vi "MainFGV.vi"(7 "FGV_mods":T1, 8 "Error In":errorcluster, 11 "DataIn":variant) -> (0 "Error Out":errorcluster, 3 "DataOut":variant)   [LabVIEW 2016]
uses:
  MainFGV_mods.ctl
  Log/log_mods.ctl
  Log/log_status.ctl
  <vilib>/DAQmx/read.llb/DAQmx Read (Analog 2D DBL NChan NSamp).vi
  <vilib>/DAQmx/miscellaneous.llb/DAQmx Fill In Error Info.vi
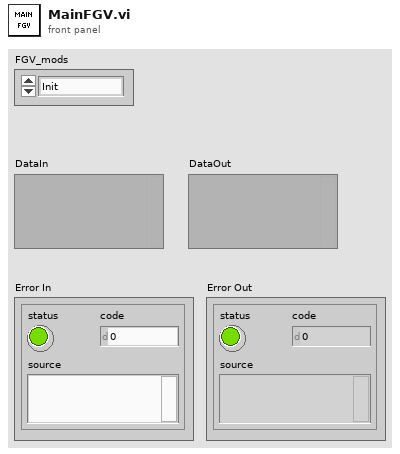
[diagram p1: front panel]
types:
  T1 = typedef "MainFGV_mods.ctl" = enum16{"Init", "Config", "Advanced", "CreateTask", "Register", "Acquire", "Start", "Burst", "Record", "End"}
  T2 = typedef "log_mods.ctl" = enum16{"Init", "LogFileRefnum", "SetStatus", "WriteAcel", "WriteToLog", "End"}
  T3 = typedef "log_status.ctl" = enum16{"Init", "Ready", "Running", "Error", "End"}
  T4 = typedef "MainFGV_data.ctl" = cluster{"TestDir":path, "TestName":string, "task":refnum<k21>, "data_file":refnum<file>, "burts_file":refnum<file>, "log_file":refnum<file>, "SamplesPerChannel":dbl, "AcqQueue":refnum<queue>, "StartTime":timestamp, "config_channels":T5[], "DAQmx Device":tag, "Advanced":T6}
  T5 = typedef "config_board.ctl" = cluster{"Sens 1":dbl, "active 1":bool, "type 1":bool, "type 2":bool, "active 2":bool, "Sens 2":dbl, "type 3":bool, "active 3":bool, "Sens 3":dbl, "type 4":bool, "active 4":bool, "Sens 4":dbl}
  T6 = typedef "AdvancedConfig.ctl" = cluster{"rate":dbl, "duration":dbl, "thr":dbl, "preTrigger":dbl, "cutoff":dbl, "Filtro":enum16{"Desativado", "Passa banda", "Passa alta", "Passa baixa"}, "highPass":dbl, "lowPass":dbl}
  T7 = cluster{"seconds since 1Jan1904":timestamp, dbl[]}
  T8 = cluster{"seconds since 1Jan1904":timestamp, dbl[][]}
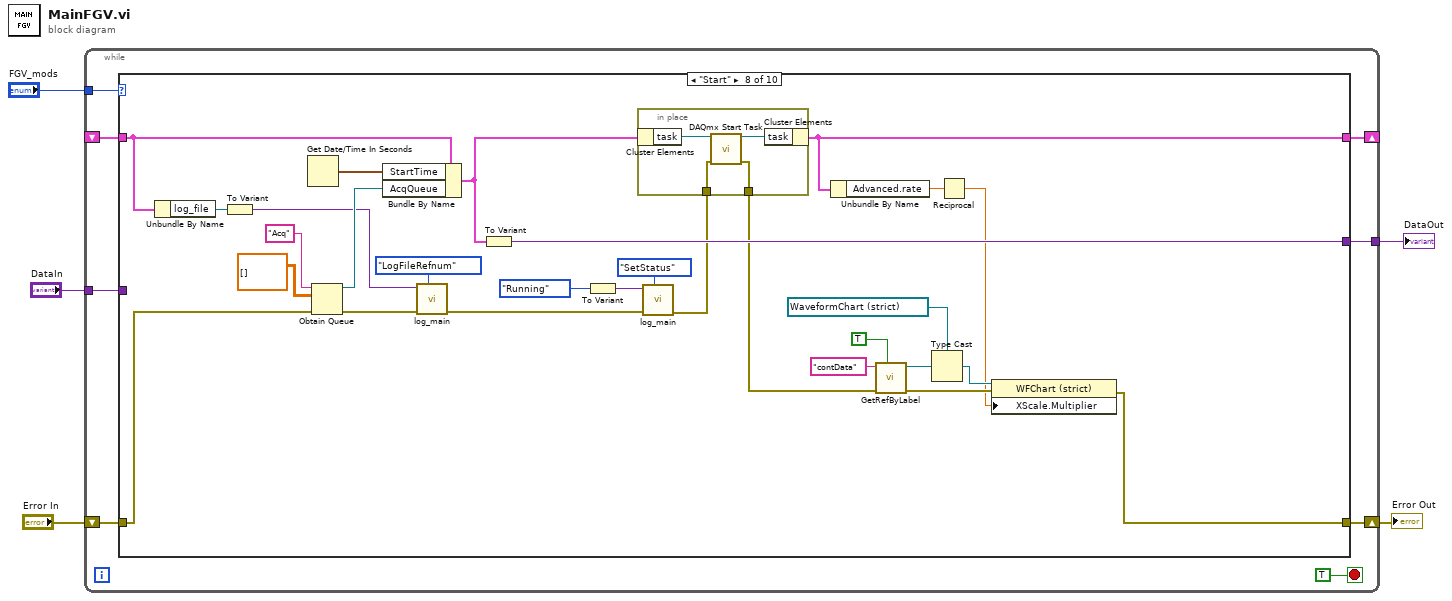
[diagram p0: block diagram]
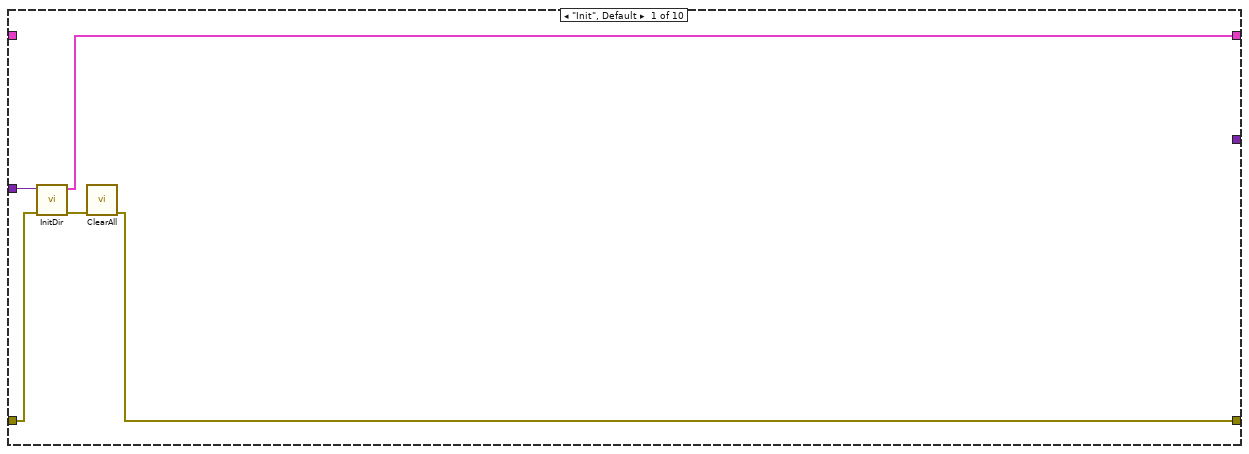
[diagram p2: hidden frame]
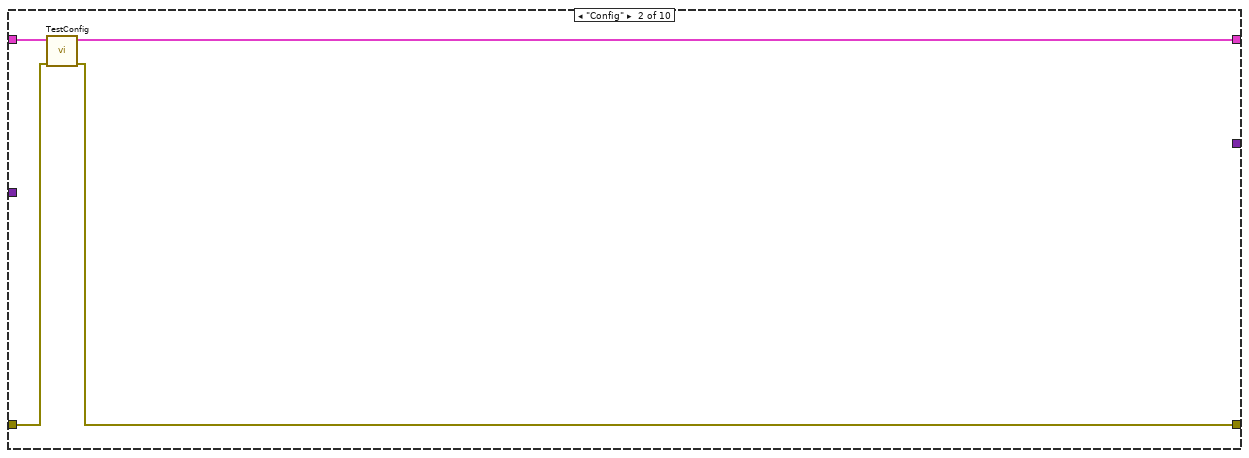
[diagram p3: hidden frame]
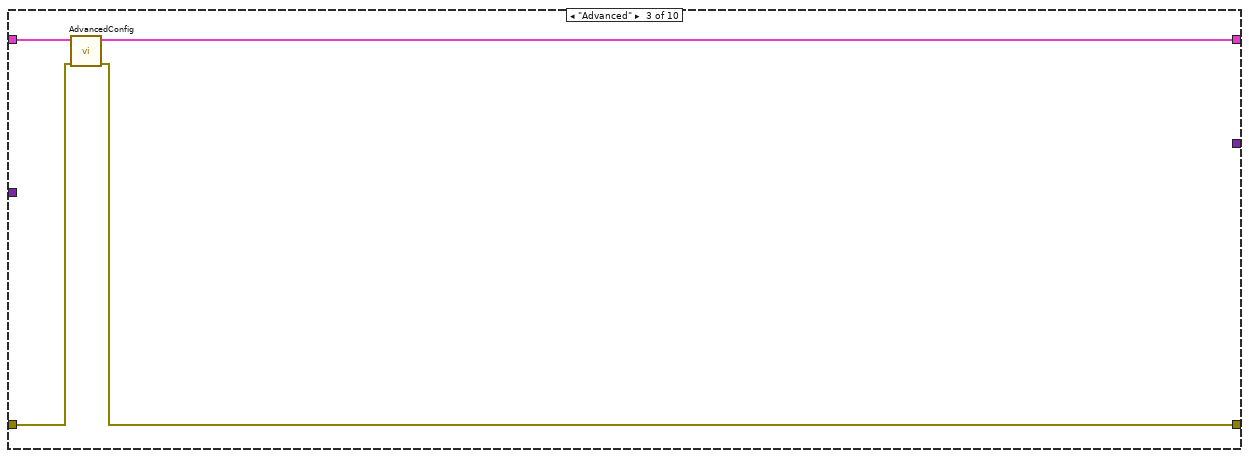
[diagram p4: hidden frame]
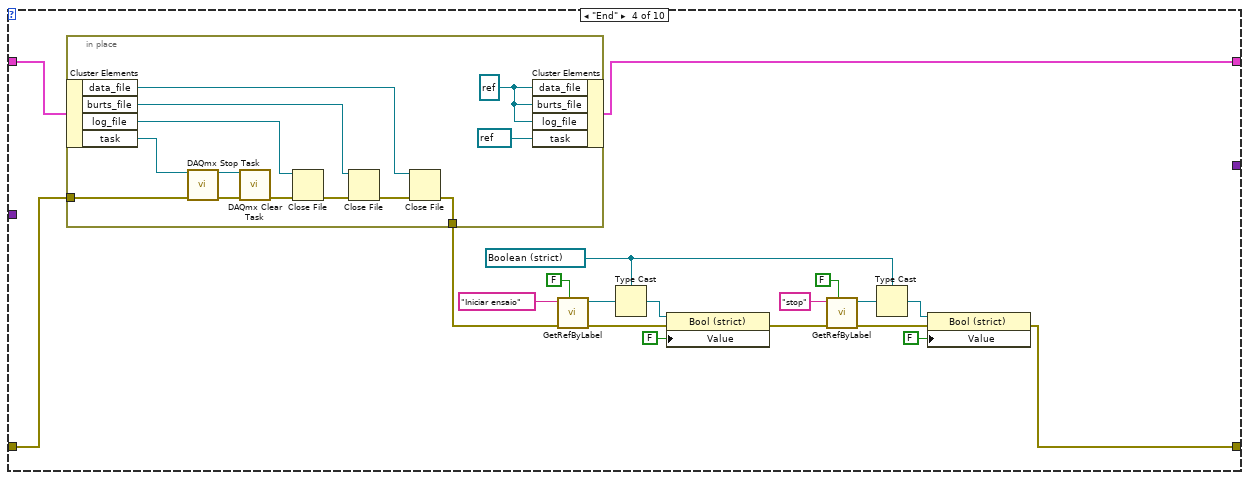
[diagram p5: hidden frame]
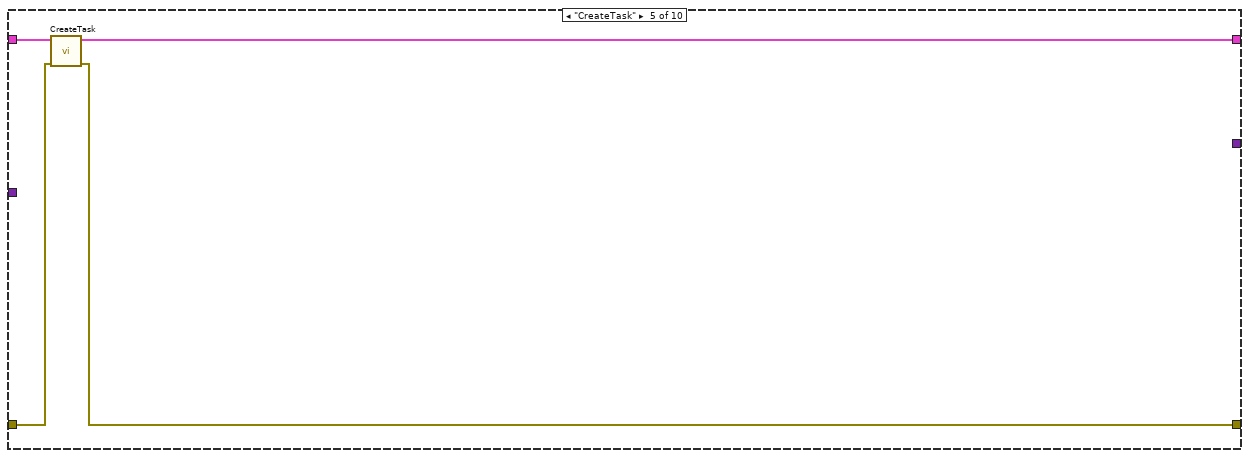
[diagram p6: hidden frame]
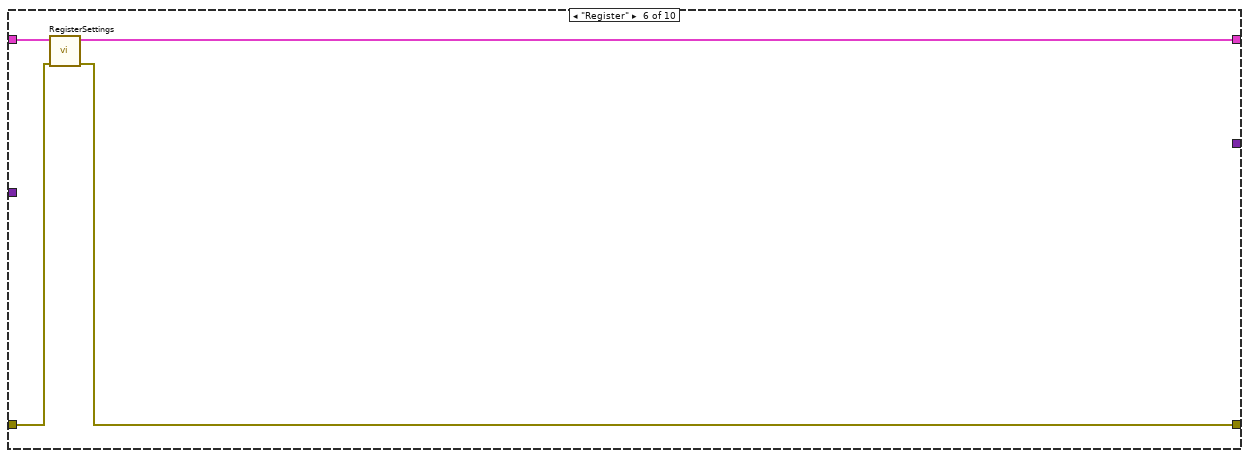
[diagram p7: hidden frame]
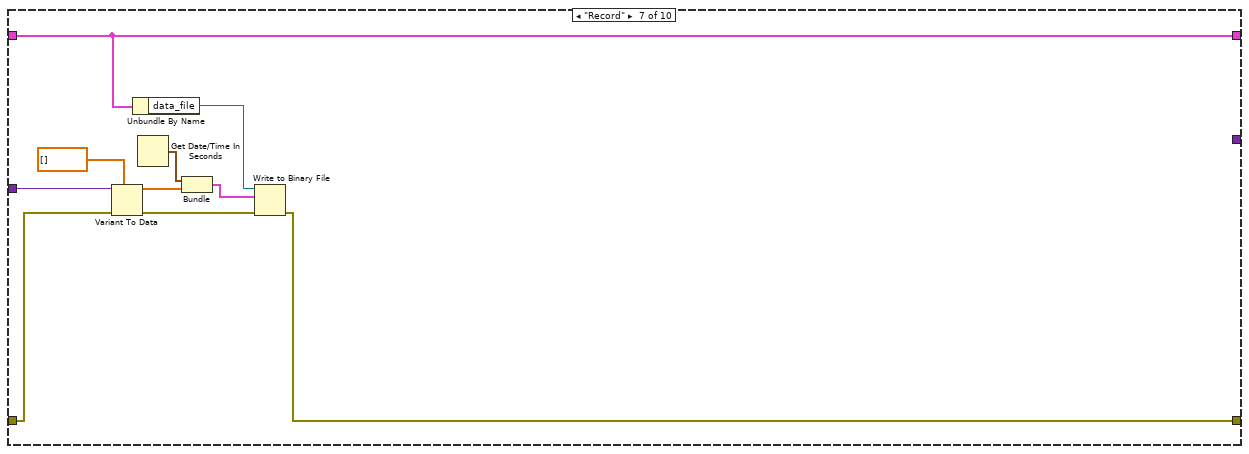
[diagram p8: hidden frame]
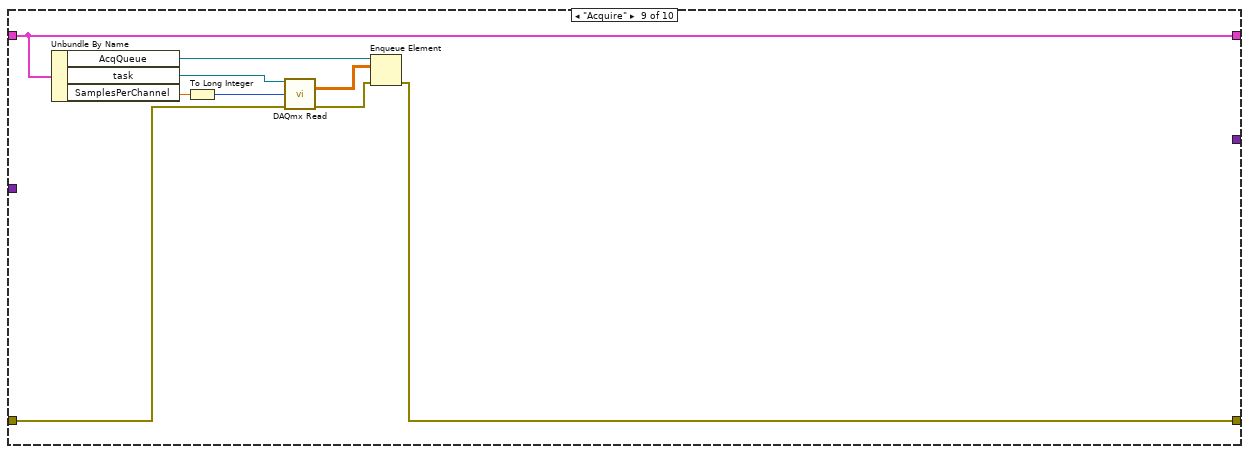
[diagram p9: hidden frame]
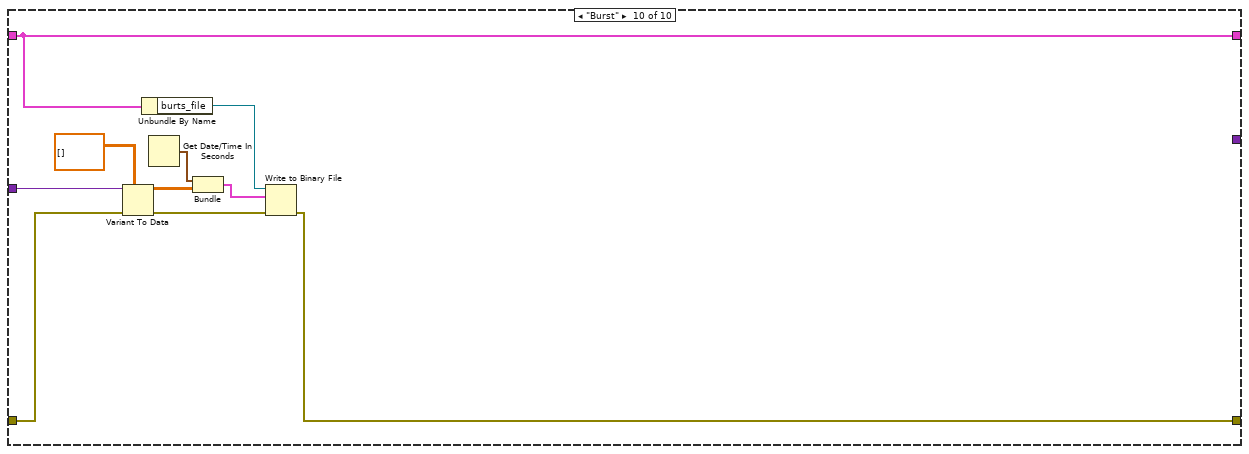
[diagram p10: hidden frame]
diagram:
  n1 = while {
    tunnel: "DataIn" -> [w12]
    tunnel: "FGV_mods" -> [w11]
    shift-right: [w10] -> _
    shift-left: _ -> [w9]
    shift-right: [w7] -> w2
    shift-left: "Error In" -> [w8]
    tunnel: [w6] -> w1
    stop <- TRUE stop-if-true
    n2 = case shown="\"Start\"" w11 {
      tunnel: w12 -> [w18 _ _ _ _ _ w76 _ _ w121]
      tunnel: [w16 w20 w25 w43 w59 w65 w71 w79 w116 w119] -> w10
      tunnel: w9 -> [_ w22 w26 w45 w62 w66 w71 w89 w116 w119]
      tunnel: w8 -> [w17 w21 w24 w44 w61 w64 w75 w91 w117 w120]
      tunnel: [w14 w19 w23 w27 w60 w63 w67 w80 w111 w118] -> w7
      tunnel: [_ _ _ _ _ _ _ w104 _ _] -> w6
      frame "Init", Default {
        n3 = call "InitDir.vi"("error in"=w17, "DataIn"=w18) -> ("error out"=w15:errorcluster, "MainFGV_data"=w16:T4)  [unwired: 8 in]
        n4 = call "ClearAll.vi"("error in"=w15) -> ("error out"=w14:errorcluster)  [unwired: 10 in]
      }
      frame "Config" {
        n5 = call "TestConfig.vi"("error in"=w21, "MainFGV_data"=w22) -> ("error out"=w19:errorcluster, "MainFGV_data out"=w20:T4)  [unwired: 8 in]
      }
      frame "Advanced" {
        n6 = call "AdvancedConfig.vi"("error in"=w24, "MainFGV_data"=w26) -> ("error out"=w23:errorcluster, "MainFGV_data out"=w25:T4)  [unwired: 8 in]
      }
      frame "End" {
        w29 = refnum<vi> refnum ("Iniciar ensaio")
        n7 = in-place {
          in-place-border: w44 -> [w57]
          in-place-border: [w48] -> w41
          w47 = refnum<file> refnum ("data_file")
          n8 = in-place-cluster #1(w45) -> ("data_file"=w49:refnum<file>, "burts_file"=w50:refnum<file>, "log_file"=w54:refnum<file>, "task"=w58:refnum<k21>)
          n9 = call <vilib>:"DAQmx Stop Task.vi"("task/channels in"=w58, "error in"=w57) -> ("task out"=w56:refnum<k21>, "error out"=w55:errorcluster)  [unwired: 12 in]
          n10 = call <vilib>:"DAQmx Clear Task.vi"("task in"=w56, "error in"=w55) -> ("error out"=w53:errorcluster)  [unwired: 13 in]
          n11 = Close File(refnum=w54, error in=w53) -> (error out=w52:errorcluster)  [unwired: 1 out]
          n12 = Close File(refnum=w50, error in=w52) -> (error out=w51:errorcluster)  [unwired: 1 out]
          n13 = Close File(refnum=w49, error in=w51) -> (error out=w48:errorcluster)  [unwired: 1 out]
          n14 = in-place-cluster #1("data_file"=w47, "burts_file"=w47, "log_file"=w47, "task"=refnum<k21> refnum) -> (w43:T4)
        }
        n15 = call "GetRefByLabel.vi"("InsideTab"=FALSE, "error in"=w41, "Label"="Iniciar ensaio") -> ("error out"=w35:errorcluster, "Ctl Refnum"=w37:refnum<vi>)  [unwired: 6 in, 1 out]
        n16 = Type Cast(type=w29, x=w37) -> (*(type *) &x=w36:refnum<vi>)
        n17 = property class="Bool (strict)"(reference=w36, error in=w35, "Value"=FALSE) -> (error out=w34:errorcluster)  [unwired: 1 out]
        n18 = call "GetRefByLabel.vi"("InsideTab"=FALSE, "error in"=w34, "Label"="stop") -> ("error out"=w30:errorcluster, "Ctl Refnum"=w28:refnum<vi>)  [unwired: 6 in, 1 out]
        n19 = Type Cast(type=w29, x=w28) -> (*(type *) &x=w31:refnum<vi>)
        n20 = property class="Bool (strict)"(reference=w31, error in=w30, "Value"=FALSE) -> (error out=w27:errorcluster)  [unwired: 1 out]
      }
      frame "CreateTask" {
        n21 = call "CreateTask.vi"("error in"=w61, "MainFGV_data"=w62) -> ("error out"=w60:errorcluster, "MainFGV_data out"=w59:T4)  [unwired: 8 in]
      }
      frame "Register" {
        n22 = call "RegisterSettings.vi"("error in"=w64, "MainFGV_data"=w66) -> ("error out"=w63:errorcluster, "MainFGV_data out"=w65:T4)  [unwired: 8 in]
      }
      frame "Record" {
        n23 = Variant To Data(error in=w75, type=dbl[] [], Variant=w76) -> (data=w73:dbl[], error out=w68:errorcluster)
        n24 = Unbundle By Name(w71) -> ("data_file"=w69:refnum<file>)
        n25 = Get Date/Time In Seconds() -> (seconds since 1Jan1904=w72:timestamp)
        n26 = Bundle("seconds since 1Jan1904"=w72, w73) -> (w70:T7)  [unwired: 1 in]
        n27 = Write to Binary File(file (use dialog)=w69, data=w70, error in=w68) -> (error out=w67:errorcluster)  [unwired: 3 in, 2 out]
      }
      frame "Start" {
        n28 = Unbundle By Name(w89) -> ("log_file"=w93:refnum<file>)
        n29 = To Variant(anything=w93) -> (Variant=w92:variant)
        n30 = Get Date/Time In Seconds() -> (seconds since 1Jan1904=w103:timestamp)
        n31 = Obtain Queue(name (unnamed)="Acq", element data type=dbl[][] [] ("2D array"), error in (no error)=w91) -> (queue out=w100:refnum<queue>, error out=w95:errorcluster)  [unwired: 2 in, 1 out]
        n32 = Bundle By Name(cluster=w89, "StartTime"=w103, "AcqQueue"=w100) -> (w90:T4)
        n33 = call "log_main.vi"("FGV_mods"=log_mods."LogFileRefnum", "Error In"=w95, "DataIn"=w92) -> ("Error Out"=w94:errorcluster)  [unwired: 7 in, 1 out]
        n34 = To Variant(anything=w90) -> (Variant=w104:variant)
        n35 = To Variant(anything=log_status."Running" ("log_status")) -> (Variant=w97:variant)
        n36 = call "log_main.vi"("FGV_mods"=log_mods."SetStatus", "Error In"=w94, "DataIn"=w97) -> ("Error Out"=w88:errorcluster)  [unwired: 7 in, 1 out]
        n37 = in-place {
          in-place-border: w88 -> [w107]
          in-place-border: [w106] -> w85
          n38 = in-place-cluster #2(w90) -> ("task"=w108:refnum<k21>)
          n39 = call <vilib>:"DAQmx Start Task.vi"("task/channels in"=w108, "error in"=w107) -> ("task out"=w105:refnum<k21>, "error out"=w106:errorcluster)  [unwired: 12 in]
          n40 = in-place-cluster #2("task"=w105) -> (w79:T4)
        }
        n41 = Unbundle By Name(w79) -> ("Advanced.rate"=w78:dbl)
        n42 = call "GetRefByLabel.vi"("InsideTab"=TRUE, "error in"=w85, "Label"="contData") -> ("error out"=w81:errorcluster, "Ctl Refnum"=w83:refnum<vi>)  [unwired: 6 in, 1 out]
        n43 = Type Cast(type=refnum<vi> refnum ("timeData"), x=w83) -> (*(type *) &x=w82:refnum<vi>)
        n44 = Reciprocal(x=w78) -> (1/x=w77:dbl)
        n45 = property class="WFChart (strict)"(reference=w82, error in=w81, "XScale.Multiplier"=w77) -> (error out=w80:errorcluster)  [unwired: 1 out]
      }
      frame "Acquire" {
        n46 = Unbundle By Name(w116) -> ("AcqQueue"=w114:refnum<queue>, "task"=w115:refnum<k21>, "SamplesPerChannel"=w110:dbl)
        n47 = To Long Integer(number=w110) -> (32bit integer=w109:i32)
        n48 = call-poly <vilib>:"DAQmx Read.vi"("task/channels in"=w115, "number of samples per channel"=w109, "error in"=w117) -> ("data"=w112:dbl[][], "error out"=w113:errorcluster)  [unwired: 10 in, 1 out]
        n49 = Enqueue Element(queue=w114, element=w112, error in (no error)=w113) -> (error out=w111:errorcluster)  [unwired: 1 in, 2 out]
      }
      frame "Burst" {
        n50 = Variant To Data(error in=w120, type=dbl[][] [], Variant=w121) -> (data=w126:dbl[][], error out=w122:errorcluster)
        n51 = Unbundle By Name(w119) -> ("burts_file"=w123:refnum<file>)
        n52 = Get Date/Time In Seconds() -> (seconds since 1Jan1904=w125:timestamp)
        n53 = Bundle("seconds since 1Jan1904"=w125, w126) -> (w124:T8)  [unwired: 1 in]
        n54 = Write to Binary File(file (use dialog)=w123, data=w124, error in=w122) -> (error out=w118:errorcluster)  [unwired: 3 in, 2 out]
      }
    }
  }
  "DataOut" <- w1
  "Error Out" <- w2
